vi "speedCheck.vi"() -> ()   [LabVIEW 2018]
panel:
  out "SPEED":dbl(knob) scale=0.0..25.5
  out "String to Array":string[](array[string])
  out "In Range?":bool
  out "Press next":dbl
  out "element":string
  out "Numeric":i32
  out "Array":dbl[](array[numeric])
  in  "write buffer":string="®\b"
  in  "VISA resource name":refnum<visa-resource-name>
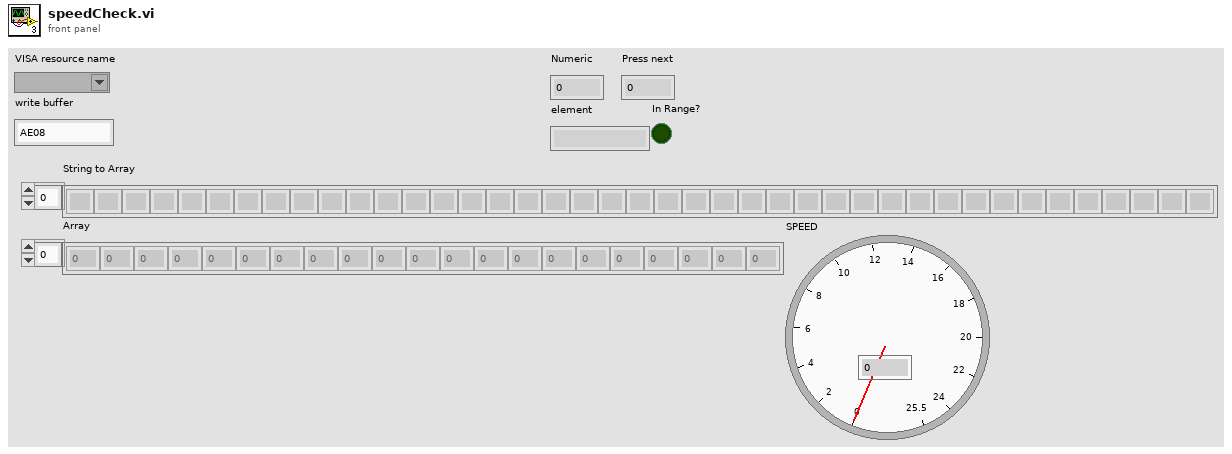
[diagram p1: front panel]
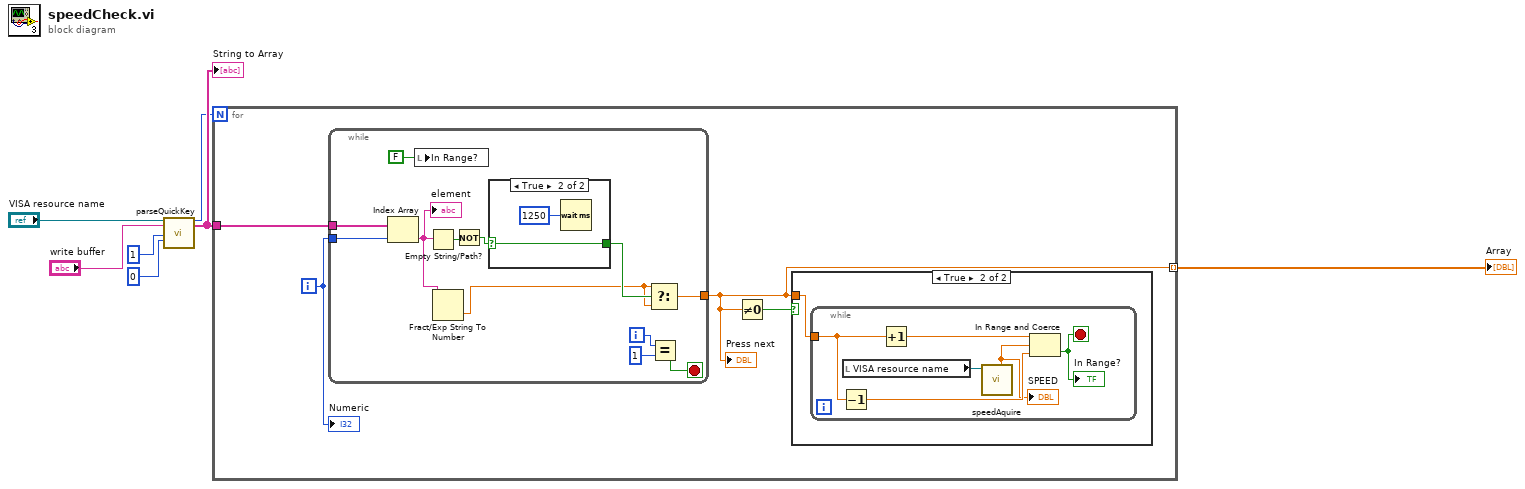
[diagram p0: block diagram]
diagram:
  n1 = call "parseQuickKey.vi"("VISA resource name"="VISA resource name", "write buffer"="write buffer", "y"=1, "x"=0) -> ("lengthString"=w1:i32, "KeyCodeName"=w2:string[])  [unwired: 11 in, 3 out]
  "String to Array" <- w2
  n2 = for {
    N: w1 -> [_]
    tunnel: w2 -> [w11]
    tunnel: [w8] -> w6 mode=indexing
    i -> [w10]
    n3 = while {
      tunnel: w11 -> [w30]
      tunnel: [w29] -> w8
      tunnel: w10 -> [w28]
      i -> [w25]
      stop <- w26 stop-if-true
      n4 = Index Array(array=w30, index=w28) -> (element=w20:string)
      "element" <- w20
      n5 = local write "In Range?"(FALSE ("In Range?")) -> ()
      n6 = Empty String/Path?(string/path=w20) -> (empty?=w22:bool)
      n7 = Fract/Exp String To Number(string=w20) -> (number=w19:dbl)  [unwired: 3 in, 1 out]
      n8 = Not(x=w22) -> (.not. x?=w21:bool)
      n9 = case shown="True" w21 {
        selector: w21 -> [w31 w32]
        tunnel: [w31 w32] -> w23
        frame False {
        }
        frame True {
          n10 = Wait (ms)(milliseconds to wait=u32 1250) -> ()  [unwired: 1 out]
        }
      }
      n11 = Select(t=w19, s=w23, f=w19) -> (s? t:f=w29:dbl)
      n12 = Equal?(x=w25, y=1) -> (x = y?=w26:bool)
    }
    "Press next" <- w8
    n13 = Not Equal To 0?(x=w8) -> (x != 0?=w9:bool)
    n14 = case shown="True" w9 {
      tunnel: w8 -> [_ w12]
      frame False {
      }
      frame True {
        n15 = while {
          tunnel: w12 -> [w15]
          stop <- w18 stop-if-true
          n16 = Decrement(x=w15) -> (x-1=w16:dbl)
          n17 = local read "VISA resource name"() -> (w13:refnum<visa-resource-name>)
          n18 = Increment(x=w15) -> (x+1=w17:dbl)
          n19 = call "speedAquire.vi"("VISA resource name"=w13) -> ("SPEED"=w14:dbl)  [unwired: 6 in, 4 out]
          "SPEED" <- w14
          n20 = In Range and Coerce(upper limit=w17, x=w14, lower limit=w16) -> (In Range?=w18:bool)  [unwired: 1 out]
          "In Range?" <- w18
        }
      }
    }
    "Numeric" <- w10
  }
  "Array" <- w6
